vi "Bring Window Forward_LV2012_NI Verified.vi"() -> ()   [LabVIEW 2024]
doc: "This VI will programmatically move a window to the front whether its a LabVIEW window or not."
uses:
  Windows/System32/user32.dll
panel:
  out "error out":errorcluster
  out "Error":i32
  in  "stop":bool
  out "Handle":dbl
  in  "Go":bool
  in  "Window Name":string
  # "Overview: This VI will programmatically move a window to the front whether its a LabVIEW window or not.\nRequirements: LabVIEW 2012 (or compatible)\nInstructions: \n1. Choose the window name you want to bring to front\n2. Run the VI\n3. Stop Execution"
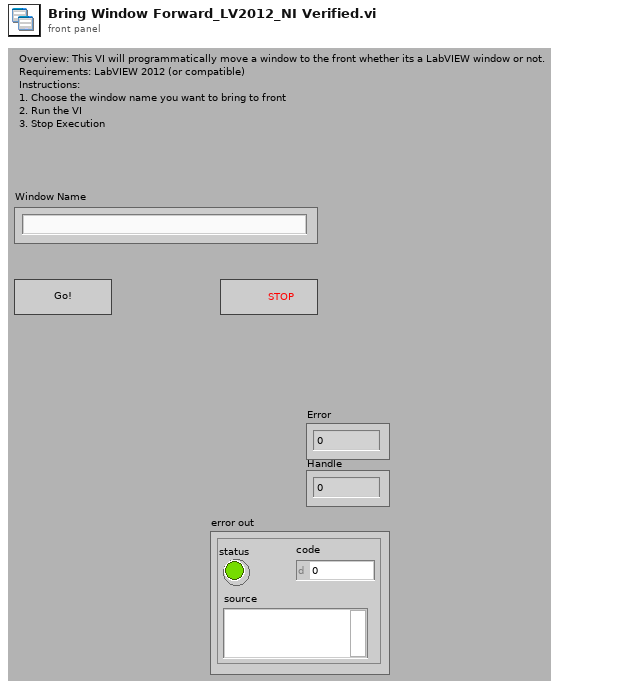
[diagram p1: front panel]
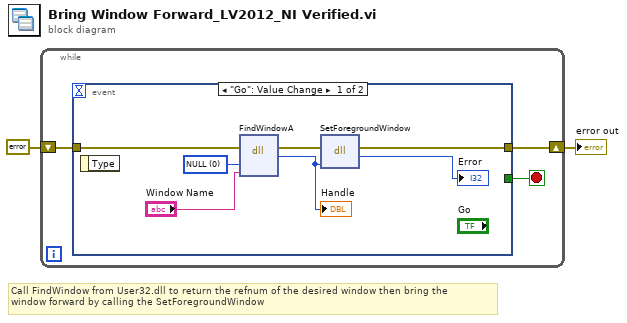
[diagram p0: block diagram]
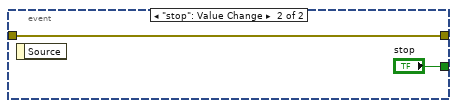
[diagram p2: hidden frame]
diagram:
  # "Call FindWindow from User32.dll to return the refnum of the desired window then bring the \nwindow forward by calling the SetForegroundWindow"
  n1 = while {
    shift-right: [w4] -> w2
    shift-left: errorcluster {"status"=FALSE, "code"=0, "source"=""} ("error out") -> [w3]
    stop <- w5 stop-if-true
    n2 = event shown="[0] \"Go\": Value Change" {
      selector: _ -> [_ _]
      dyn-events: _ -> [_ _]
      timeout: _ -> [_ _]
      tunnel: [_ "stop"] -> w5
      tunnel: [w7 w13] -> w4
      tunnel: w3 -> [w6 w13]
      event "Go": Value Change {
        w12 = 0 items=["NULL"]
        n3 = event-data() -> ()  [unwired: 2 out]
        n4 = dll-call lib="/Windows/System32/user32.dll" fn="FindWindowA" label="FindWindow"(error in=w6, "lpszClassName"=w12, "lpszWindowName"="Window Name") -> (error out=w8:errorcluster, "hWnd"=w10:u32)  [unwired: 3 in, 2 out]
        "Handle" <- w10
        n5 = dll-call lib="/Windows/System32/user32.dll" fn="SetForegroundWindow"(error in=w8, "Handle"=w10) -> (error out=w7:errorcluster, "return type"=→"Error":i32)  [unwired: 3 in, 1 out]
      }
      event "stop": Value Change {
        n6 = event-data() -> ()  [unwired: 2 out]
      }
    }
  }
  "error out" <- w2
